vi "CASE STRUCTURE WITH NUMERIC.vi"() -> ()   [LabVIEW 2018]
panel:
  in  "Dial":i8(knob) scale=0.0..10.0
  out "RESULT":dbl
  in  "Y":dbl
  in  "X":dbl
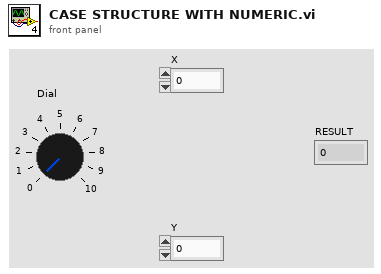
[diagram p1: front panel]
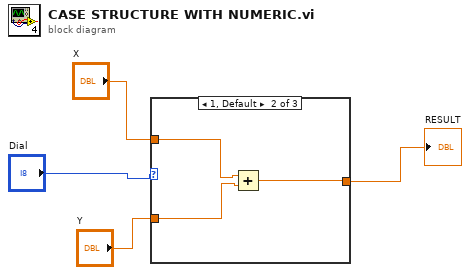
[diagram p0: block diagram]
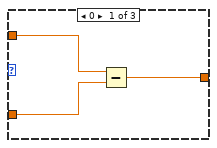
[diagram p2: hidden frame]
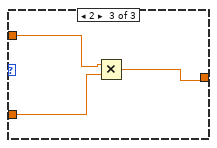
[diagram p3: hidden frame]
diagram:
  n1 = case shown="1, Default" "Dial" {
    tunnel: "X" -> [w7 w9 w13]
    tunnel: "Y" -> [w6 w10 w12]
    tunnel: [w5 w8 w11] -> w2
    frame 0 {
      n2 = Subtract(x=w7, y=w6) -> (x-y=w5:dbl)
    }
    frame 1, Default {
      n3 = Add(x=w9, y=w10) -> (x+y=w8:dbl)
    }
    frame 2 {
      n4 = Multiply(x=w13, y=w12) -> (x*y=w11:dbl)
    }
  }
  "RESULT" <- w2
